vi "Cross_Correlate.vi"(4 "Time window half width":dbl, 6 "interp. method":i32(ring) items=["nearest", "linear", "spline", "cubic Hermite", "Lagrange"], 7 "Shift input array":dbl[](array[numeric]) format="%.2f", 8 "Time Cluster 2":T1, 9 "Time Cluster 1":T1, 10 "Cluster 2":T2={"Colour"=0, "Inst type"=enum."Pitot-static tube", "Inst name"="Manometer voltage", "Symbol"="U", "Code name"="", "Extra Info"="U", "Inst Array"=enum."PWA", "Extra Titles"=[], "Extra Values"=[], "U"=0.0, "u^2"=0.0, "u^3"=0.0, "u^4"=0.0, "Skew_u"=0.0, "Kurt_u"=0.0, "Sd Error in Mean"=0.0, "% u'/U"=0.0, "X"=0.0, "Y"=0.0, "Z"=0.0, "Timescale integral to 25%"=0.0, "Sd Error in Variance"=0.0, "Calib File"=path "", "Calib Constants"=[], "Output Position"=FALSE, "Full Stats"=FALSE, "Av Sampling Rate"=0.0, "Av No of Samples"=0.0, "Total Meas Time (s)"=0.0, "ADAM Ch Name"=""} {"Sd Error in Variance" format="%.2f"; "Skew_u" format="%.2f"; "% u'/U" format="%.2f"; "Sd Error in Mean" format="%.2f"; "Kurt_u" format="%.2f"; "u^4" format="%.2f"; "u^3" format="%.2f"; "U" format="%.2f"; "u^2" format="%.2f"}, 11 "Cluster 1":T2={"Colour"=0, "Inst type"=enum."Pitot-static tube", "Inst name"="Manometer voltage", "Symbol"="U", "Code name"="", "Extra Info"="U", "Inst Array"=enum."PWA", "Extra Titles"=[], "Extra Values"=[], "U"=0.0, "u^2"=0.0, "u^3"=0.0, "u^4"=0.0, "Skew_u"=0.0, "Kurt_u"=0.0, "Sd Error in Mean"=0.0, "% u'/U"=0.0, "X"=0.0, "Y"=0.0, "Z"=0.0, "Timescale integral to 25%"=0.0, "Sd Error in Variance"=0.0, "Calib File"=path "", "Calib Constants"=[], "Output Position"=FALSE, "Full Stats"=FALSE, "Av Sampling Rate"=0.0, "Av No of Samples"=0.0, "Total Meas Time (s)"=0.0, "ADAM Ch Name"=""} {"Sd Error in Variance" format="%.2f"; "Skew_u" format="%.2f"; "% u'/U" format="%.2f"; "Sd Error in Mean" format="%.2f"; "Kurt_u" format="%.2f"; "u^4" format="%.2f"; "u^3" format="%.2f"; "U" format="%.2f"; "u^2" format="%.2f"}) -> (0 "Plug In Values":string[](array[string]), 1 "Plug In Titles":string[](array[string]), 2 "XY Graph":cluster{dbl[], dbl[]}(graph), 3 "Shift output array":dbl[](array[numeric]) format="%.2f")   [LabVIEW 2013]
uses:
  Controls/Analysis_info_cluster.ctl
  Controls/Inst_type.ctl
  Controls/Instrument_Array.ctl
  Controls/Time_Trace_Cluster.ctl
  Globals/Meas_global.vi
  <vilib>/Analysis/2dsp.llb/1D Cross Correlation (DBL).vi
  <vilib>/gmath/NI_Gmath.lvlib
  <vilib>/Analysis/NI_AALPro.lvlib
  <vilib>/Analysis/NI_AALBase.lvlib
panel:
  out "Time(s) for Max":dbl
  out "Max Corr Coeff":dbl
  out "Av Sampling Rate":dbl
  out "Equi spaced":bool
  out "Times match":bool
  out "Start Time":dbl
  out "End Time":dbl
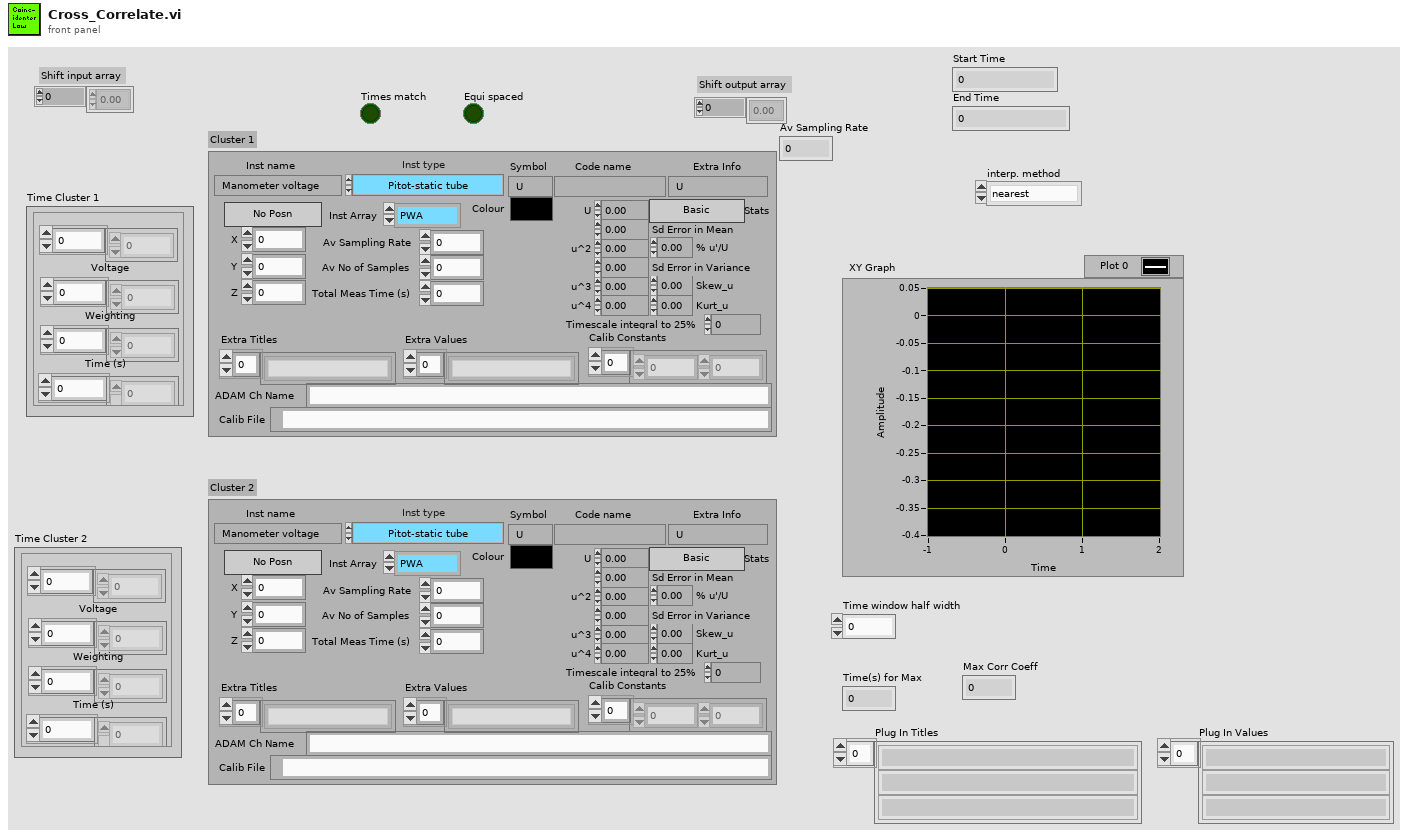
[diagram p1: front panel]
types:
  T1 = typedef "Time_Trace_Cluster.ctl" = cluster{"Weighting":dbl[], "Time (s)":dbl[], "Voltage":dbl[], "Eng Values":dbl[]}
  T2 = typedef "Analysis_info_cluster.ctl" = cluster{"Colour":u32, "Inst type":T3, "Inst name":string, "Symbol":string, "Code name":string, "Extra Info":string, "Inst Array":T4, "Extra Titles":string[], "Extra Values":string[], "U":dbl, "u^2":dbl, "u^3":dbl, "u^4":dbl, "Skew_u":dbl, "Kurt_u":dbl, "Sd Error in Mean":dbl, "% u'/U":dbl, "X":dbl, "Y":dbl, "Z":dbl, "Timescale integral to 25%":dbl, "Sd Error in Variance":dbl, "Calib File":path, "Calib Constants":dbl[], "Output Position":bool, "Full Stats":bool, "Av Sampling Rate":dbl, "Av No of Samples":dbl, "Total Meas Time (s)":dbl, "ADAM Ch Name":string}
  T3 = typedef "Inst_type.ctl" = enum16{"Propeller anemometer", "Raw voltage", "Pressure Transducer", "Pitot-static tube", "Preston tube", "Hot wire", "Cross wire 1", "Cross wire 2", "Generic Linear", "Generic Polynomial", "Generic BackPoly", "Fast FID", "Thermocouple", "Cold wire", "Pulsed Wire", "LDA Vel", "LDA Tran time", "LDA Arr time"}
  T4 = typedef "Instrument_Array.ctl" = enum16{"PWA", "LDA", "Analogue"}
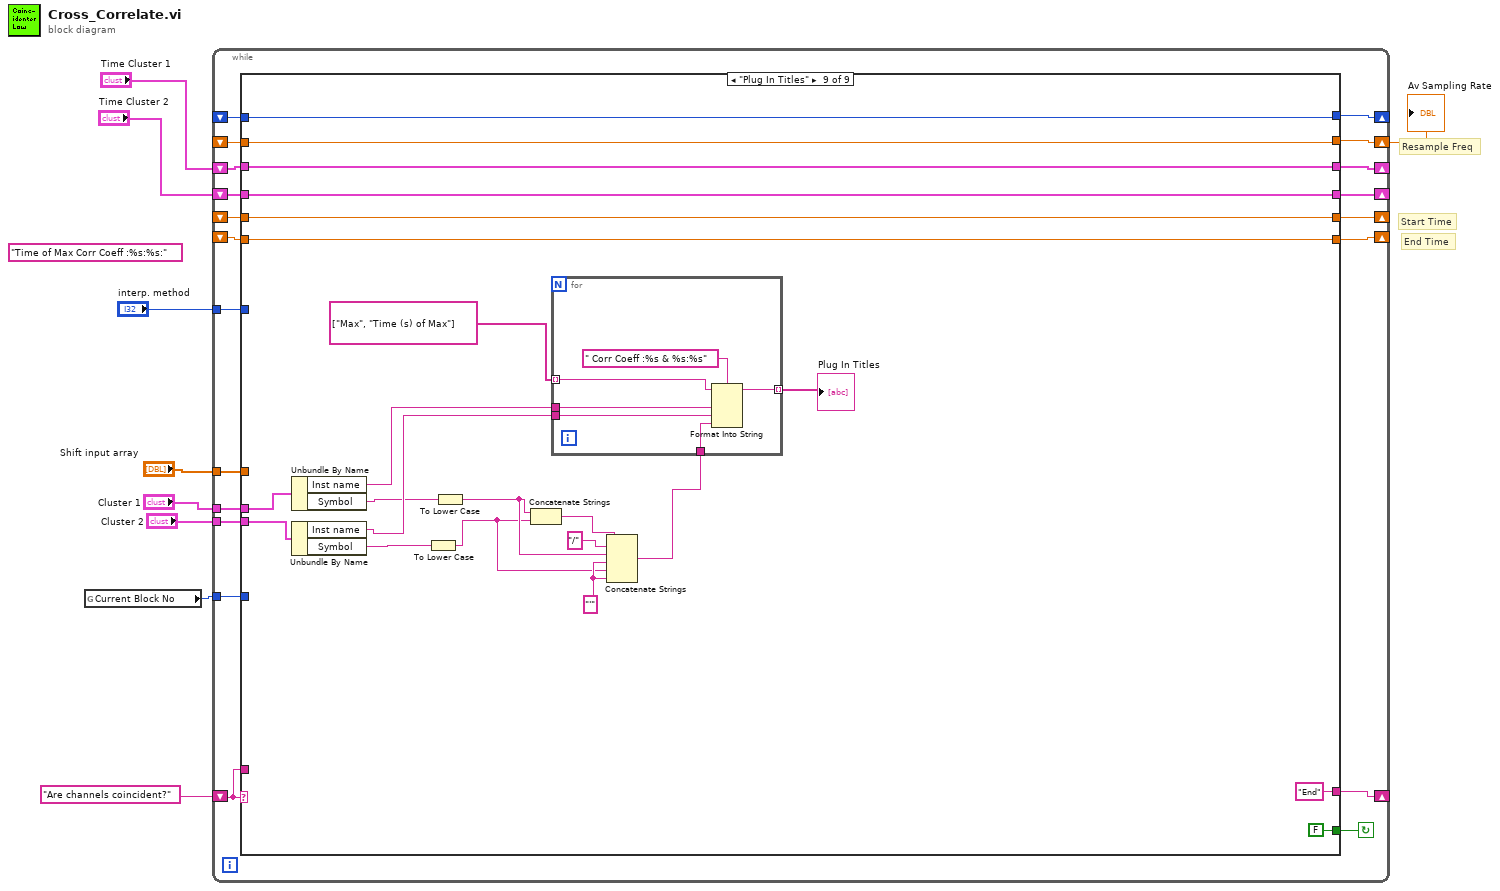
[diagram p0: block diagram]
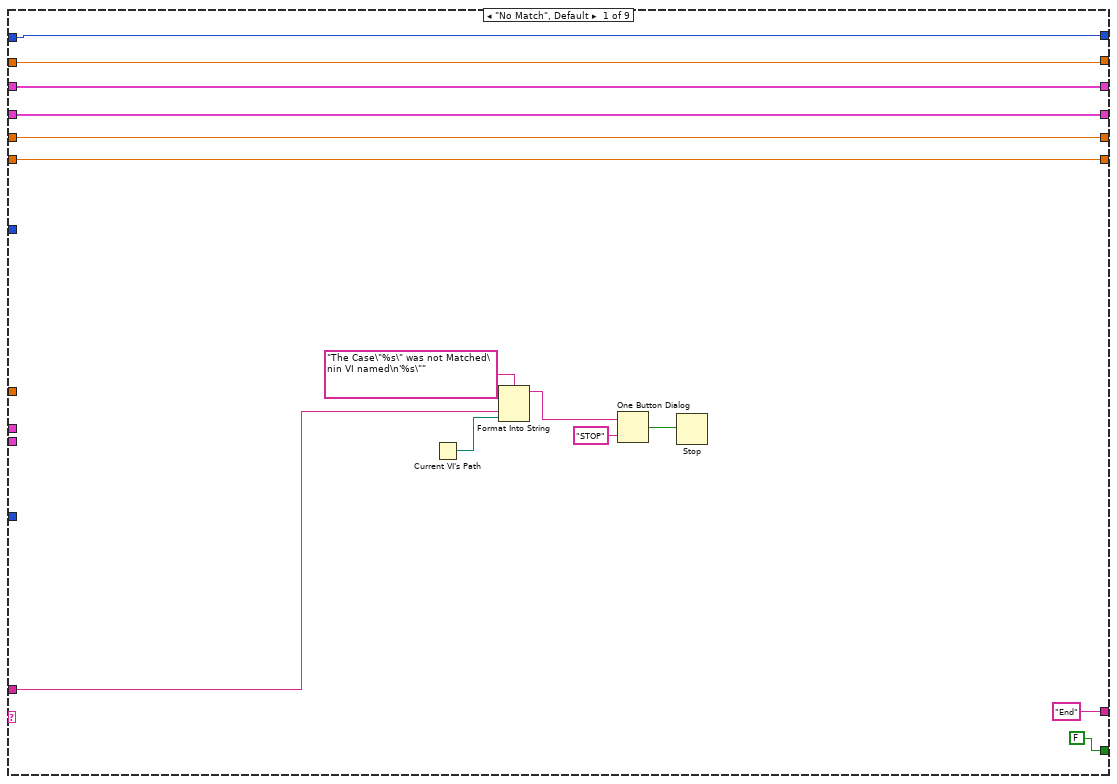
[diagram p2: hidden frame]
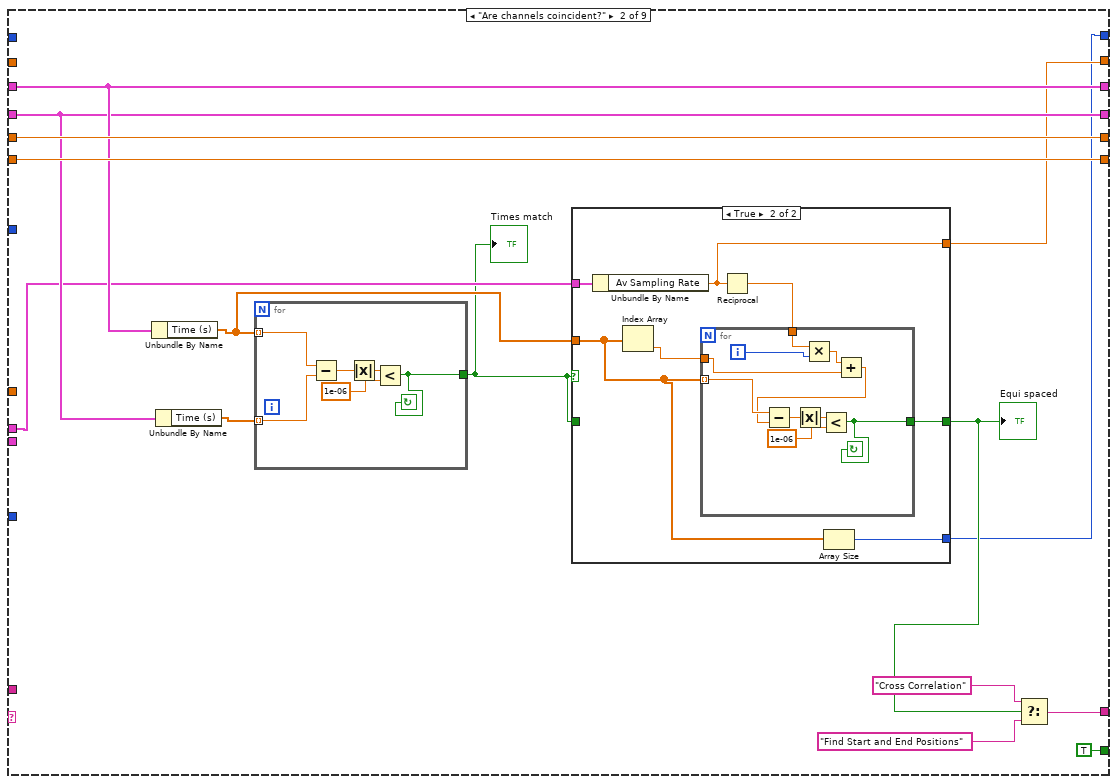
[diagram p3: hidden frame]
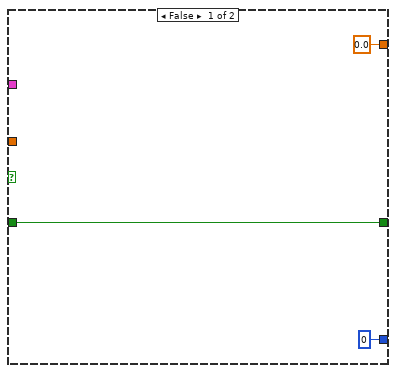
[diagram p4: hidden frame]
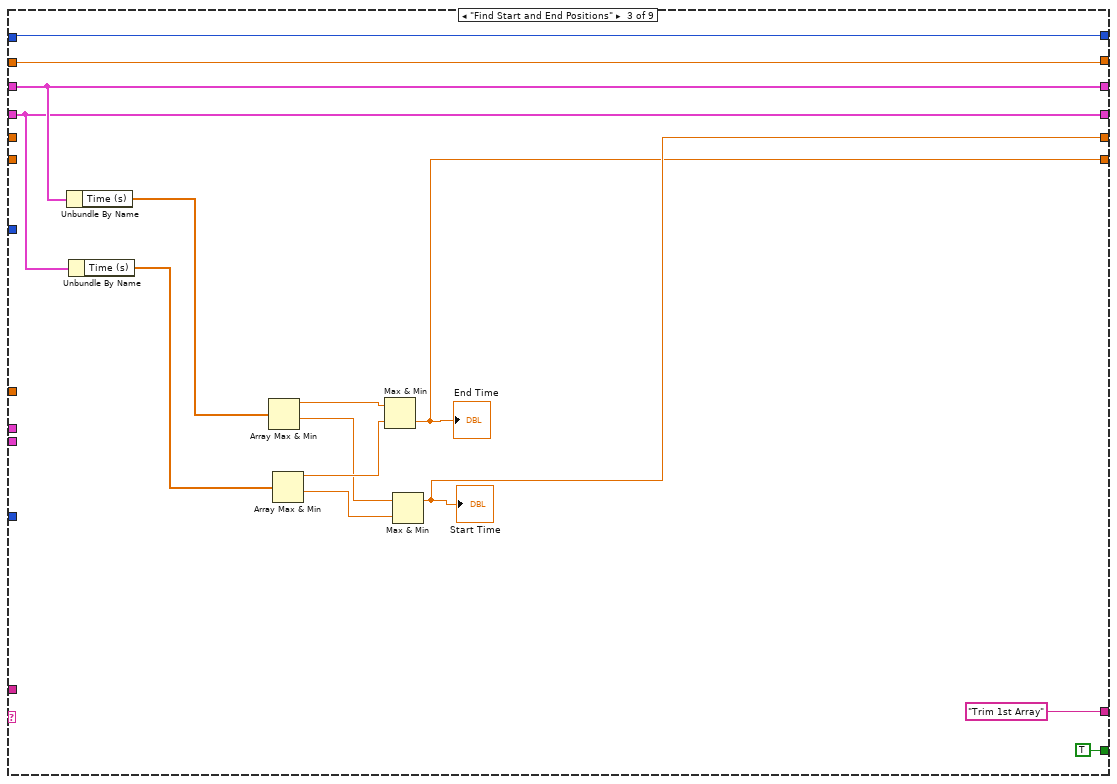
[diagram p5: hidden frame]
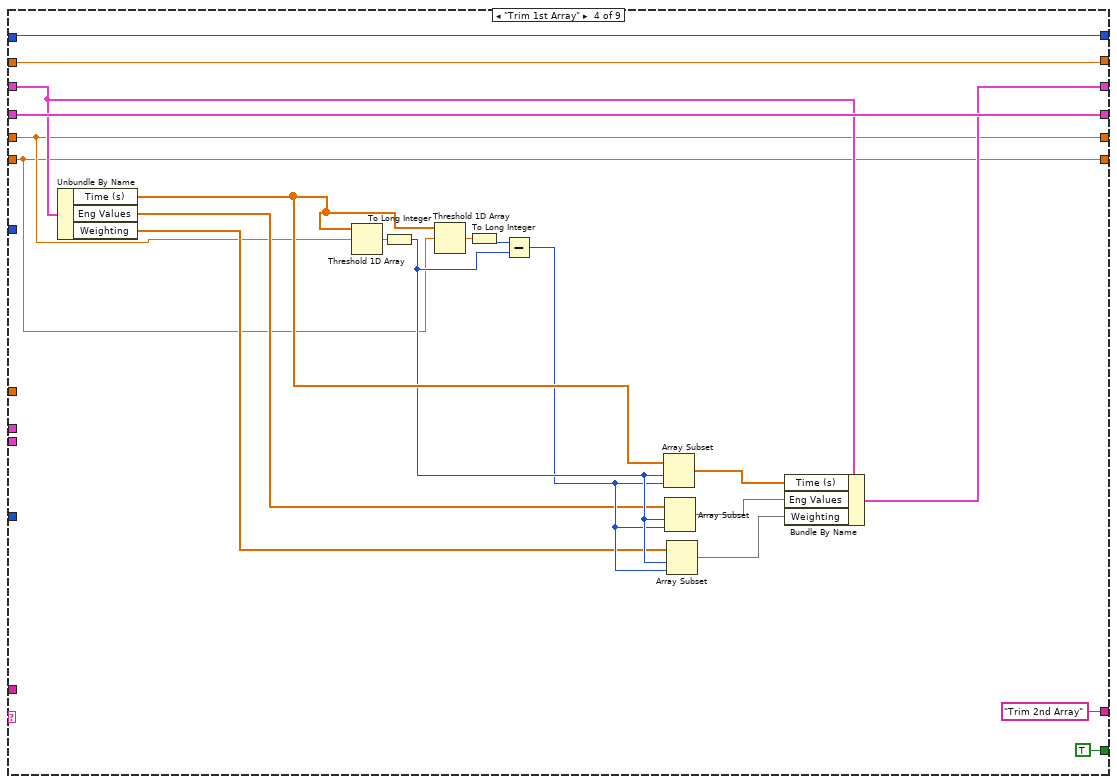
[diagram p6: hidden frame]
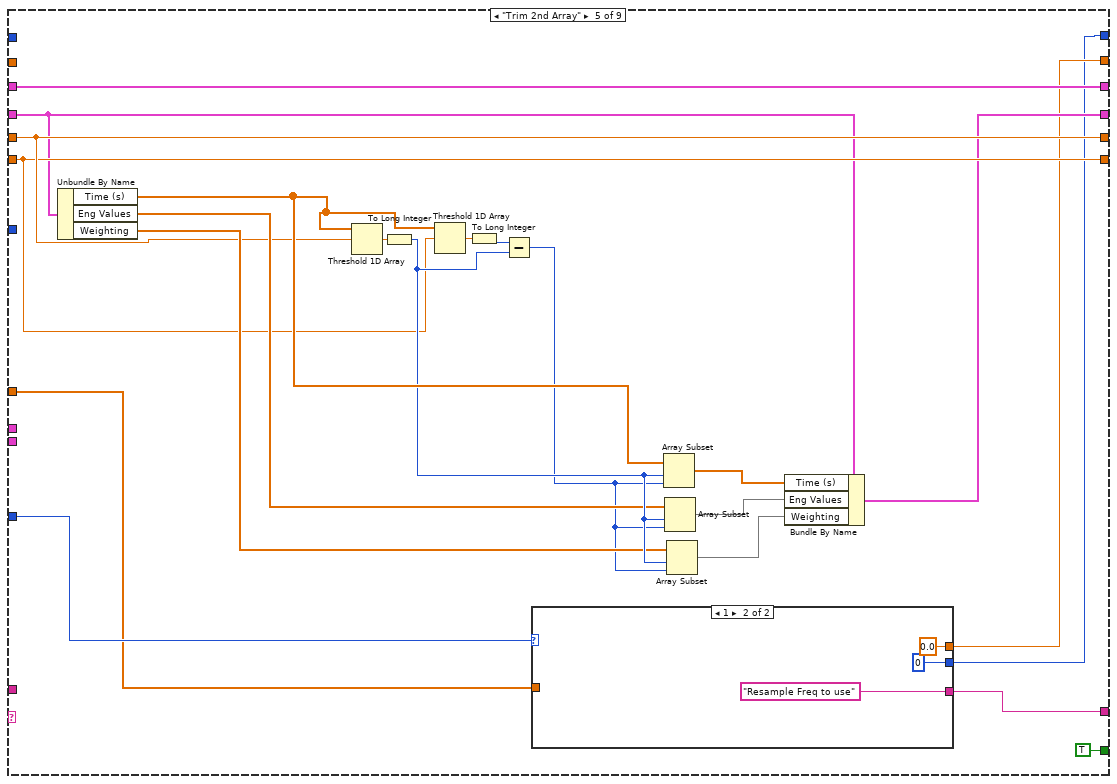
[diagram p7: hidden frame]
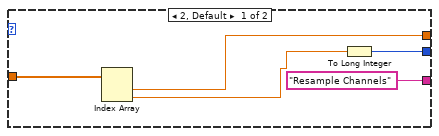
[diagram p8: hidden frame]
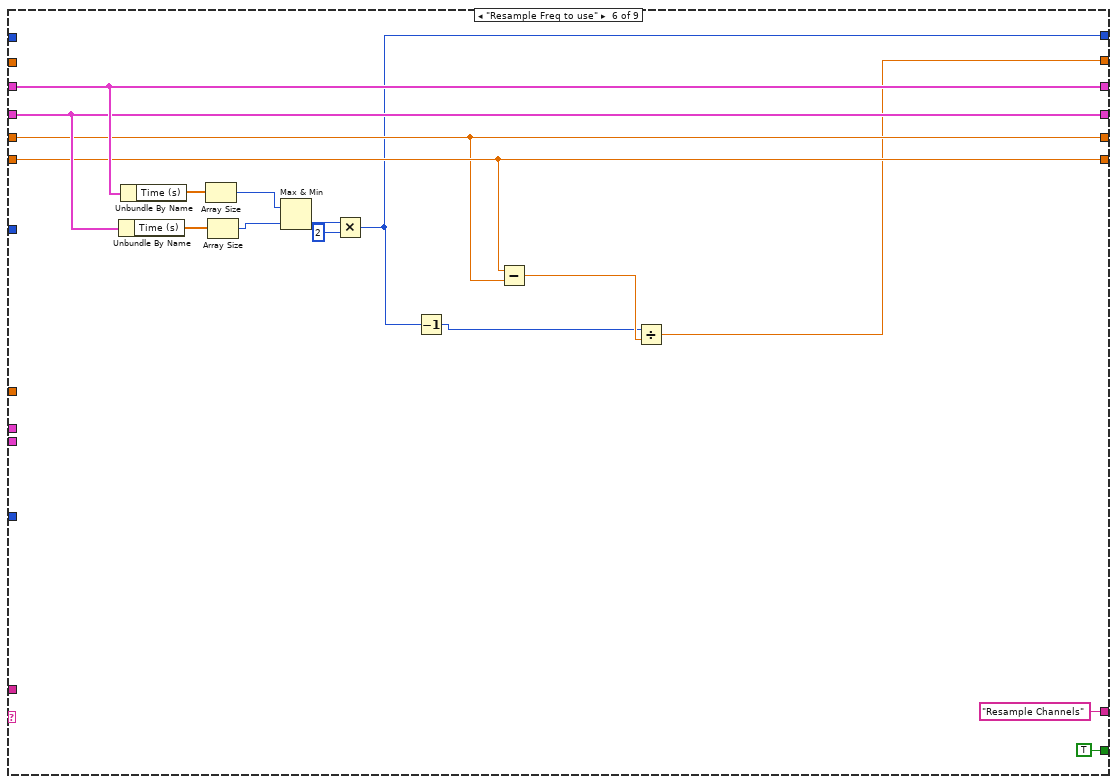
[diagram p9: hidden frame]
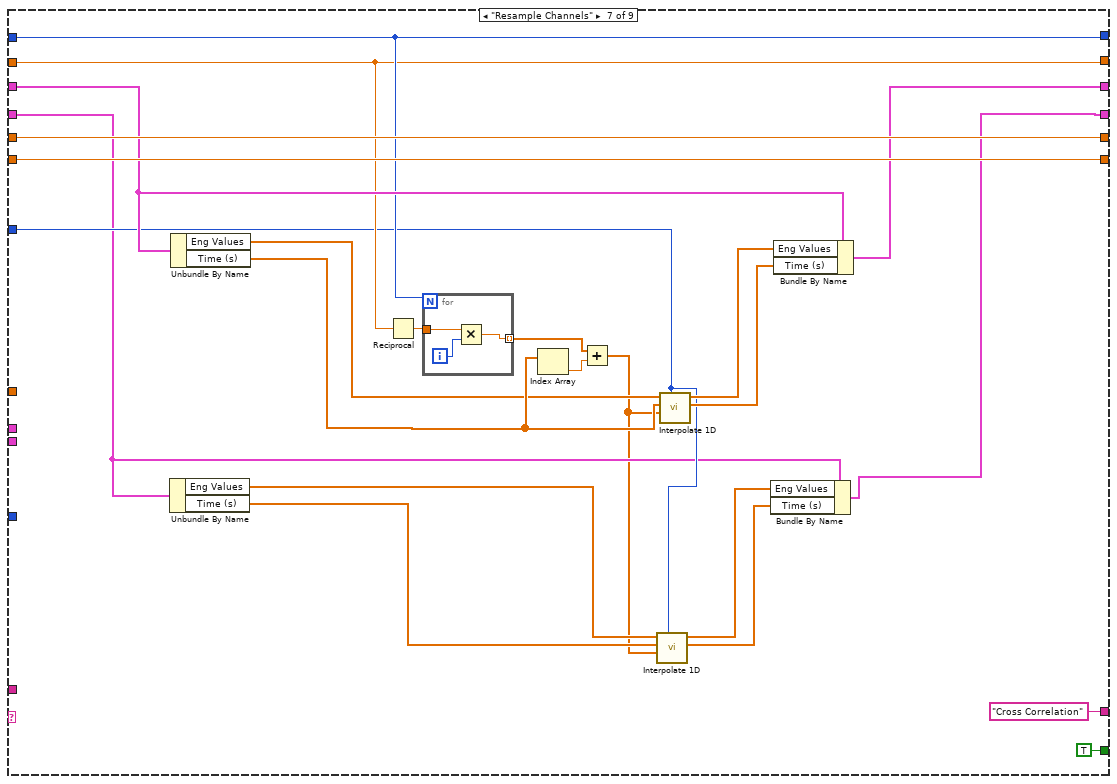
[diagram p10: hidden frame]
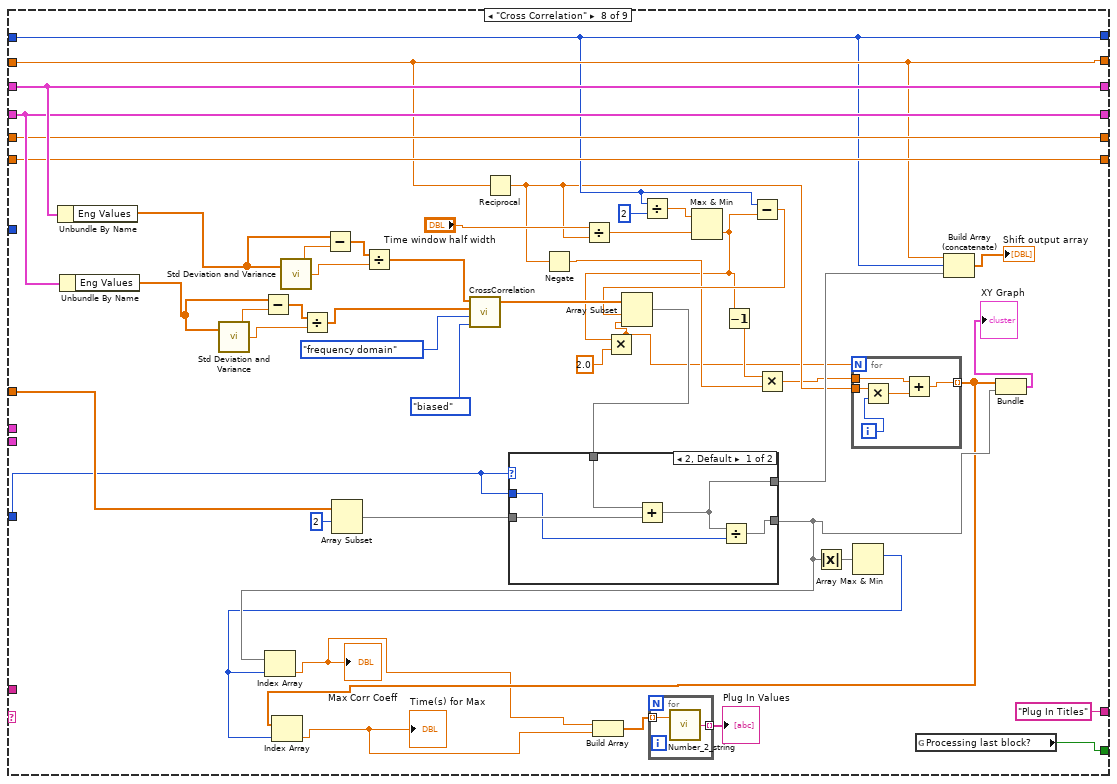
[diagram p11: hidden frame]
diagram:
  (unwired) "Time of Max Corr Coeff :%s:%s:" ("format string")
  # "Resample Freq"
  # "End Time"
  # "Start Time"
  n1 = global read "Meas_global.vi" "Current Block No"() -> (w5:i32)
  n2 = while {
    shift-right: [w24] -> _
    shift-left: "Time Cluster 1" -> [w26]
    shift-right: [w23] -> _
    shift-left: "Time Cluster 2" -> [w25]
    shift-right: [w27] -> _
    shift-left: "Are channels coincident?" -> [w29]
    shift-right: [w21] -> _
    shift-left: _ -> [w22]
    shift-right: [w20] -> _
    shift-left: _ -> [w19]
    tunnel: "interp. method" -> [w18]
    tunnel: "Cluster 1" -> [w17]
    tunnel: "Cluster 2" -> [w16]
    shift-right: [w13] -> w1
    shift-left: _ -> [w12]
    tunnel: w5 -> [w15]
    tunnel: "Shift input array" -> [w14]
    shift-right: [w10] -> _
    shift-left: _ -> [w11]
    stop <- w28 continue-if-true
    n3 = case shown="\"Plug In Titles\"" w29 {
      tunnel: w29 -> [w38 _ _ _ _ _ _ _ _]
      tunnel: [FALSE TRUE ("Show Plots") TRUE TRUE TRUE TRUE ("Show Plots") TRUE ("Show Plots") w195 FALSE ("Processing last block?")] -> w28
      tunnel: ["End" w48 "Trim 1st Array" "Trim 2nd Array" w122 "Resample Channels" ("t") "Cross Correlation" "Plug In Titles" ("t") "End" ("t")] -> w27
      tunnel: w26 -> [w35 w56 w97 w114 w126 w164 w184 w239 w274]
      tunnel: w25 -> [w34 w55 w96 w117 w127 w163 w169 w238 w273]
      tunnel: [w35 w56 w97 w104 w126 w164 w185 w239 w274] -> w24
      tunnel: [w34 w55 w96 w117 w128 w163 w168 w238 w273] -> w23
      tunnel: w22 -> [w33 w58 _ w103 w130 w157 w187 w237 w272]
      tunnel: [w33 w58 w89 w103 w130 w157 w187 w237 w272] -> w21
      tunnel: [w32 w57 w88 w102 w129 w158 w186 w236 w271] -> w20
      tunnel: w19 -> [w32 w57 _ w102 w129 w158 w186 w236 w271]
      tunnel: w18 -> [_ _ _ _ _ _ w170 _ _]
      tunnel: w17 -> [_ w53 _ _ _ _ _ _ w266]
      tunnel: w16 -> [_ _ _ _ _ _ _ _ w265]
      tunnel: w15 -> [_ _ _ _ w123 _ _ w217 _]
      tunnel: w14 -> [_ _ _ _ w121 _ _ w221 _]
      tunnel: [w31 w45 w87 w100 w120 w156 w179 w216 w270] -> w13
      tunnel: w12 -> [w31 _ w87 w100 _ _ w179 w216 w270]
      tunnel: [w30 w44 w86 w99 w119 w149 w180 w208 w269] -> w10
      tunnel: w11 -> [w30 _ w86 w99 _ _ w180 w208 w269]
      frame "No Match", Default {
        n4 = Current VI's Path() -> (path=w43:path)
        n5 = Format Into String(format string="The Case\"%s\" was not Matched\nin VI named\n'%s\"" ("Format String"), w38, w43) -> (resulting string=w40:string)  [unwired: 2 in, 1 out]
        n6 = One Button Dialog(message=w40, button name ("OK")="STOP") -> (true=w42:bool)
        n7 = Stop(stop? (T)=w42) -> ()
      }
      frame "Are channels coincident?" {
        n8 = Unbundle By Name(w56) -> ("Time (s)"=w52:dbl[])
        n9 = Unbundle By Name(w55) -> ("Time (s)"=w54:dbl[])
        n10 = for {
          tunnel: w52 -> [w80] mode=indexing
          tunnel: w54 -> [w81] mode=indexing
          tunnel: [w79] -> w51
          stop <- w79 continue-if-true
          n11 = Subtract(x=w80, y=w81) -> (x-y=w84:dbl)
          n12 = Absolute Value(x=w84) -> (abs(x)=w83:dbl)
          n13 = Less?(x=w83, y=1e-06) -> (x < y?=w79:bool)
        }
        "Times match" <- w51
        n14 = case shown="True" w51 {
          tunnel: w53 -> [_ w68]
          tunnel: w52 -> [_ w64]
          tunnel: [w61 w67] -> w50
          tunnel: w51 -> [w61 _]
          tunnel: [0.0 ("Av Sampling Rate") w65] -> w45
          tunnel: [0 w63] -> w44
          frame False {
          }
          frame True {
            n15 = Unbundle By Name(w68) -> ("Av Sampling Rate"=w65:dbl)
            n16 = Index Array(array=w64) -> (element=w66:dbl)  [unwired: 1 in]
            n17 = Reciprocal(x=w65) -> (1/x=w62:dbl)
            n18 = for {
              tunnel: w64 -> [w75] mode=indexing
              tunnel: [w74] -> w67
              tunnel: w62 -> [w73]
              tunnel: w66 -> [w70]
              i -> [w71]
              stop <- w74 continue-if-true
              n19 = Multiply(x=w73, y=w71) -> (x*y=w72:dbl)
              n20 = Add(x=w72, y=w70) -> (x+y=w69:dbl)
              n21 = Subtract(x=w75, y=w69) -> (x-y=w78:dbl)
              n22 = Absolute Value(x=w78) -> (abs(x)=w77:dbl)
              n23 = Less?(x=w77, y=1e-06) -> (x < y?=w74:bool)
            }
            n24 = Array Size(array=w64) -> (size(s)=w63:i32)
          }
        }
        "Equi spaced" <- w50
        n25 = Select(t="Cross Correlation", s=w50, f="Find Start and End Positions") -> (s? t:f=w48:string)
      }
      frame "Find Start and End Positions" {
        n26 = Unbundle By Name(w97) -> ("Time (s)"=w90:dbl[])
        n27 = Unbundle By Name(w96) -> ("Time (s)"=w95:dbl[])
        n28 = Array Max & Min(array=w90) -> (max value=w94:dbl, min value=w92:dbl)  [unwired: 2 out]
        n29 = Array Max & Min(array=w95) -> (max value=w93:dbl, min value=w91:dbl)  [unwired: 2 out]
        n30 = Max & Min(x=w94, y=w93) -> (min(x,y)=w88:dbl)  [unwired: 1 out]
        "End Time" <- w88
        n31 = Max & Min(x=w92, y=w91) -> (max(x,y)=w89:dbl)  [unwired: 1 out]
        "Start Time" <- w89
      }
      frame "Trim 1st Array" {
        n32 = Unbundle By Name(w114) -> ("Time (s)"=w113:dbl[], "Eng Values"=w109:dbl[], "Weighting"=w108:dbl[])
        n33 = Threshold 1D Array(2:w103, 3:w113) -> (0:w115:dbl)  [unwired: 1 in]
        n34 = To Long Integer(number=w115) -> (32bit integer=w111:i32)
        n35 = Threshold 1D Array(2:w102, 3:w113) -> (0:w116:dbl)  [unwired: 1 in]
        n36 = To Long Integer(number=w116) -> (32bit integer=w112:i32)
        n37 = Subtract(x=w112, y=w111) -> (x-y=w110:i32)
        n38 = Array Subset(array=w113, index=w111, length=w110) -> (w107:dbl[])
        n39 = Array Subset(array=w109, index=w111, length=w110) -> (w106:dbl[])
        n40 = Array Subset(array=w108, index=w111, length=w110) -> (w105:dbl[])
        n41 = Bundle By Name(cluster=w114, "Time (s)"=w107, "Eng Values"=w106, "Weighting"=w105) -> (w104:T1)
      }
      frame "Trim 2nd Array" {
        n42 = Unbundle By Name(w127) -> ("Time (s)"=w137:dbl[], "Eng Values"=w134:dbl[], "Weighting"=w133:dbl[])
        n43 = Threshold 1D Array(2:w130, 3:w137) -> (0:w138:dbl)  [unwired: 1 in]
        n44 = To Long Integer(number=w138) -> (32bit integer=w135:i32)
        n45 = Threshold 1D Array(2:w129, 3:w137) -> (0:w139:dbl)  [unwired: 1 in]
        n46 = To Long Integer(number=w139) -> (32bit integer=w136:i32)
        n47 = Subtract(x=w136, y=w135) -> (x-y=w125:i32)
        n48 = case shown="1" w123 {
          tunnel: ["Resample Channels" ("t") "Resample Freq to use"] -> w122
          tunnel: w121 -> [w145 _]
          tunnel: [w144 0.0] -> w120
          tunnel: [w141 0] -> w119
          frame 2, Default {
            n49 = Index Array(array=w145) -> (element #1=w144:dbl, element #2=w142:dbl)  [unwired: 2 in]
            n50 = To Long Integer(number=w142) -> (32bit integer=w141:i32)
          }
          frame 1 {
          }
        }
        n51 = Array Subset(array=w137, index=w135, length=w125) -> (w124:dbl[])
        n52 = Array Subset(array=w134, index=w135, length=w125) -> (w132:dbl[])
        n53 = Array Subset(array=w133, index=w135, length=w125) -> (w131:dbl[])
        n54 = Bundle By Name(cluster=w127, "Time (s)"=w124, "Eng Values"=w132, "Weighting"=w131) -> (w128:T1)
      }
      frame "Resample Freq to use" {
        n55 = Unbundle By Name(w163) -> ("Time (s)"=w161:dbl[])
        n56 = Unbundle By Name(w164) -> ("Time (s)"=w162:dbl[])
        n57 = Array Size(array=w162) -> (size(s)=w159:i32)
        n58 = Array Size(array=w161) -> (size(s)=w160:i32)
        n59 = Max & Min(x=w159, y=w160) -> (min(x,y)=w151:i32)  [unwired: 1 out]
        n60 = Multiply(x=w151, y=2) -> (x*y=w149:i32)
        n61 = Decrement(x=w149) -> (x-1=w152:i32)
        n62 = Subtract(x=w158, y=w157) -> (x-y=w153:dbl)
        n63 = Divide(x=w152, y=w153) -> (x/y=w156:dbl)
      }
      frame "Resample Channels" {
        n64 = Unbundle By Name(w169) -> ("Eng Values"=w172:dbl[], "Time (s)"=w171:dbl[])
        n65 = Unbundle By Name(w184) -> ("Eng Values"=w177:dbl[], "Time (s)"=w178:dbl[])
        n66 = Reciprocal(x=w179) -> (1/x=w182:dbl)
        n67 = for {
          N: w180 -> [_]
          tunnel: w182 -> [w190]
          tunnel: [w188] -> w167 mode=indexing
          i -> [w189]
          n68 = Multiply(x=w190, y=w189) -> (x*y=w188:dbl)
        }
        n69 = Index Array(array=w178) -> (element=w181:dbl)  [unwired: 1 in]
        n70 = Add(x=w167, y=w181) -> (x+y=w166:dbl[])
        n71 = call <vilib>:"Interpolate 1D.vi"("method"=w170, "xi"=w166, "X"=w171, "Y"=w172) -> ("xi used"=w174:dbl[], "yi"=w173:dbl[])  [unwired: 2 in, 4 out]
        n72 = call <vilib>:"Interpolate 1D.vi"("method"=w170, "xi"=w166, "X"=w178, "Y"=w177) -> ("xi used"=w175:dbl[], "yi"=w176:dbl[])  [unwired: 2 in, 4 out]
        n73 = Bundle By Name(cluster=w169, "Eng Values"=w173, "Time (s)"=w174) -> (w168:T1)
        n74 = Bundle By Name(cluster=w184, "Eng Values"=w176, "Time (s)"=w175) -> (w185:T1)
      }
      frame "Cross Correlation" {
        n75 = Unbundle By Name(w239) -> ("Eng Values"=w231:dbl[])
        n76 = Unbundle By Name(w238) -> ("Eng Values"=w223:dbl[])
        n77 = call <vilib>:"Std Deviation and Variance.vi"("X"=w223) -> ("mean"=w224:dbl, "standard deviation"=w226:dbl)  [unwired: 1 in, 1 out]
        n78 = Subtract(x=w223, y=w224) -> (x-y=w225:dbl[])
        n79 = call <vilib>:"Std Deviation and Variance.vi"("X"=w231) -> ("mean"=w230:dbl, "standard deviation"=w228:dbl)  [unwired: 1 in, 1 out]
        n80 = Divide(x=w225, y=w226) -> (x/y=w222:dbl[])
        n81 = Subtract(x=w231, y=w230) -> (x-y=w229:dbl[])
        n82 = Array Subset(array=w221, index=2) -> (w219:dbl[])  [unwired: 1 in]
        n83 = Divide(x=w229, y=w228) -> (x/y=w227:dbl[])
        n84 = call-poly <vilib>:"CrossCorrelation.vi"("normalization"=enum32{"none", "unbiased", "biased"}."biased", "algorithm"=enum32{"direct", "frequency domain"}."frequency domain", "Y"=w222, "X"=w227) -> ("Rxy"=w210:dbl[])  [unwired: 6 in, 1 out]
        n85 = Reciprocal(x=w216) -> (1/x=w202:dbl)
        n86 = Negate(x=w202) -> (-x=w206:dbl)
        n87 = Divide(x="Time window half width", y=w202) -> (x/y=w212:dbl)
        n88 = Divide(x=w208, y=2) -> (x/y=w213:dbl)
        n89 = Max & Min(x=w213, y=w212) -> (min(x,y)=w205:dbl)  [unwired: 1 out]
        n90 = Multiply(x=w205, y=2.0) -> (x*y=w200:dbl)
        n91 = Decrement(x=w205) -> (x-1=w204:dbl)
        n92 = Subtract(x=w208, y=w205) -> (x-y=w207:dbl)
        n93 = Array Subset(array=w210, index=w207, length=w200) -> (w209:dbl[])
        n94 = case shown="2, Default" w217 {
          tunnel: w209 -> [w251 w252]
          tunnel: w219 -> [w250 _]
          tunnel: [w247 w252] -> w199
          tunnel: [w249 w252] -> w218
          tunnel: w217 -> [w248 _]
          frame 2, Default {
            n95 = Add(x=w251, y=w250) -> (x+y=w249:dbl[])
            n96 = Divide(x=w249, y=w248) -> (x/y=w247:dbl[])
          }
          frame 1 {
          }
        }
        n97 = Multiply(x=w204, y=w206) -> (x*y=w201:dbl)
        n98 = Absolute Value(x=w199) -> (abs(x)=w203:dbl[])
        n99 = for {
          N: w200 -> [_]
          tunnel: w202 -> [w244]
          tunnel: w201 -> [w243]
          tunnel: [w242] -> w196 mode=indexing
          i -> [w245]
          n100 = Multiply(x=w244, y=w245) -> (x*y=w246:dbl)
          n101 = Add(x=w243, y=w246) -> (x+y=w242:dbl)
        }
        n102 = Array Max & Min(array=w203) -> (max index (indices)=w197:i32)  [unwired: 3 out]
        n103 = Index Array(array=w199, index=w197) -> (element=w193:dbl)
        "Max Corr Coeff" <- w193
        n104 = Index Array(array=w196, index=w197) -> (element=w192:dbl)
        "Time(s) for Max" <- w192
        n105 = Build Array(w193, w192) -> (w194:dbl[])
        n106 = for {
          tunnel: w194 -> [w240] mode=indexing
          tunnel: [w241] -> w191 mode=indexing
          n107 = call "Number_2_string.vi"("number"=w240) -> ("String"=w241:string)  [unwired: 1 in]
        }
        "Plug In Values" <- w191
        n108 = global read "Meas_global.vi" "Processing last block?"() -> (w195:bool)
        n109 = Build Array (concatenate)(w216, w208, w218) -> (→"Shift output array":dbl[])
        n110 = Bundle(w196, w199) -> (→"XY Graph":cluster{dbl[], dbl[]})  [unwired: 1 in]
      }
      frame "Plug In Titles" {
        w260 = "'"
        n111 = Unbundle By Name(w266) -> ("Inst name"=w264:string, "Symbol"=w262:string)
        n112 = Unbundle By Name(w265) -> ("Inst name"=w263:string, "Symbol"=w261:string)
        n113 = To Lower Case(string=w261) -> (all lower case string=w256:string)
        n114 = To Lower Case(string=w262) -> (all lower case string=w257:string)
        n115 = Concatenate Strings(w257, w256) -> (w258:string)
        n116 = Concatenate Strings(w258, "/", w257, w260, w256, w260) -> (w255:string)
        n117 = for {
          tunnel: w264 -> [w279]
          tunnel: w263 -> [w278]
          tunnel: w255 -> [w277]
          tunnel: string[] ["Max", "Time (s) of Max"] -> [w276] mode=indexing
          tunnel: [w275] -> w253 mode=indexing
          n118 = Format Into String(format string=" Corr Coeff :%s & %s:%s", initial string=w276, w279, w278, w277) -> (resulting string=w275:string)  [unwired: 1 in, 1 out]
        }
        "Plug In Titles" <- w253
      }
    }
  }
  "Av Sampling Rate" <- w1
